vi "HandleXMLMapping.vi"(8 "error in (no error)":errorcluster, 10 "String":string, 11 "Node Ptr":T1 format="%.0x") -> (0 "error out":errorcluster, 3 "Node Ptr Out":T1 format="%.0x")   [LabVIEW 2024, in "Embedded TDMS Logger System Explorer.lvlib"]
doc: "Given an XML description of Sources and Destinations, creates these mappings in the System Definition."
uses:
  Embedded TDMS Logger System Explorer.lvlib
  <vilib>/NI VeriStand/Custom Device API/Custom Device Item Ref.ctl
  NationalInstruments.VeriStand.SystemDefinitionAPI
  NationalInstruments.VeriStand
  <vilib>/regexp/Match Regular Expression.xnode
  <vilib>/NI VeriStand/Custom Device API/Custom Device API.lvlib
panel:
  out "Array 3":string[](array[string])
  out "Array 2":i32[](array[numeric])
  out "Array":bool[](array[boolean])
  out "AddChannelMappings":bool
  out "Destinations":string[](array[string])
  out "Sources":string[](array[string])
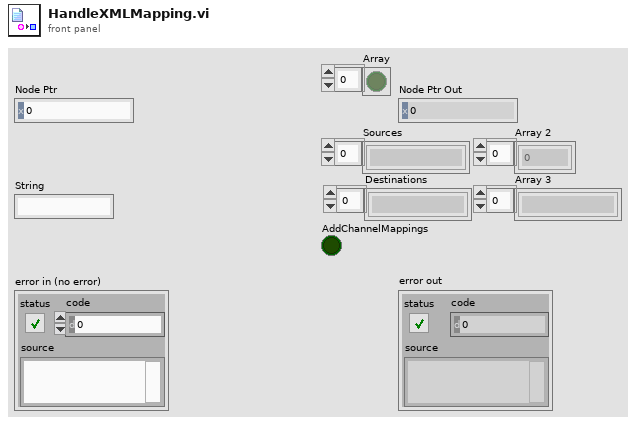
[diagram p1: front panel]
types:
  T1 = typedef "Custom Device API.lvlib/Custom Device Item Ref.ctl" = u64
  T2 = typedef "Custom Device API.lvlib/Custom Device Pointer.ctl" = refnum<k24>
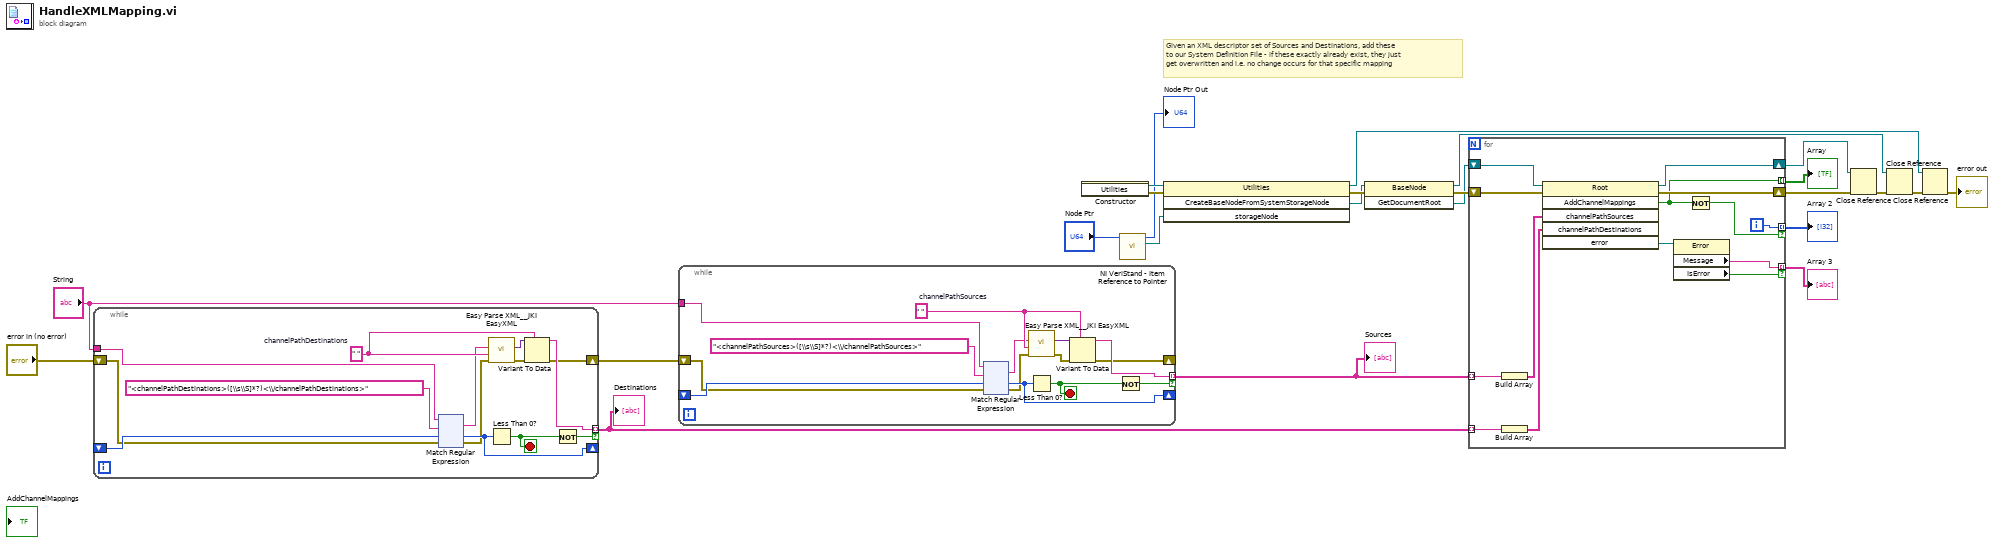
[diagram p0: block diagram]
diagram:
  # "Given an XML descriptor set of Sources and Destinations, add these\nto our System Definition File - if these exactly already exist, they just\nget overwritten and i.e. no change occurs for that specific mapping"
  n1 = while {
    shift-right: [w37] -> _
    shift-left: _ -> [w36]
    tunnel: "String" -> [w32]
    tunnel: [w31] -> w6 mode=indexing if=w28
    shift-right: [w26] -> w4
    shift-left: "error in (no error)" -> [w25]
    stop <- w27 stop-if-true
    w30 = " "  # channelPathDestinations
    n2 = xnode "Match Regular Expression"("input string"=w32, "regular expression"="<channelPathDestinations>([\\s\\S]*?)<\\/channelPathDestinations>" ("format string"), "offset (0)"=w36, "error in"=w25) -> ("whole match"=w29:string, "offset past match"=w37:i32, "error out"=w33:errorcluster)  [unwired: 2 in, 2 out]
    n3 = call <vilib>:"Easy Parse XML__JKI EasyXML.vi"("error in (no error)"=w33, "LabVIEW Data (Type)"=w30, "XML String"=w29) -> ("error out"=w35:errorcluster, "LabVIEW Data"=w34:variant)  [unwired: 7 in]
    n4 = Less Than 0?(x=w37) -> (x < 0?=w27:bool)
    n5 = Variant To Data(error in=w35, type=w30, Variant=w34) -> (data=w31:string, error out=w26:errorcluster)
    n6 = Not(x=w27) -> (.not. x?=w28:bool)
  }
  "Destinations" <- w6
  n7 = while {
    shift-right: [w168] -> _
    shift-left: _ -> [w167]
    tunnel: "String" -> [w163]
    tunnel: [w162] -> w5 mode=indexing if=w159
    shift-right: [w157] -> _
    shift-left: w4 -> [w156]
    stop <- w158 stop-if-true
    w161 = " "  # channelPathSources
    n8 = xnode "Match Regular Expression"("input string"=w163, "regular expression"="<channelPathSources>([\\s\\S]*?)<\\/channelPathSources>" ("format string"), "offset (0)"=w167, "error in"=w156) -> ("whole match"=w160:string, "offset past match"=w168:i32, "error out"=w164:errorcluster)  [unwired: 2 in, 2 out]
    n9 = call <vilib>:"Easy Parse XML__JKI EasyXML.vi"("error in (no error)"=w164, "LabVIEW Data (Type)"=w161, "XML String"=w160) -> ("error out"=w166:errorcluster, "LabVIEW Data"=w165:variant)  [unwired: 7 in]
    n10 = Less Than 0?(x=w168) -> (x < 0?=w158:bool)
    n11 = Variant To Data(error in=w166, type=w161, Variant=w165) -> (data=w162:string, error out=w157:errorcluster)
    n12 = Not(x=w158) -> (.not. x?=w159:bool)
  }
  "Sources" <- w5
  n13 = constructor class="Utilities"() -> (reference out=w12:refnum<k24>, error out=w13:errorcluster)  [unwired: 3 in, 1 out]
  n14 = call <vilib>:"NI VeriStand - Item Reference to Pointer.vi"("Item Ref in"="Node Ptr") -> ("Node Pointer"=w16:T2, "Item Ref out"=→"Node Ptr Out":T1)  [unwired: 7 in, 2 out]
  n15 = invoke class="Utilities" method="CreateBaseNodeFromSystemStorageNode"(reference=w12, error in=w13, "storageNode"=w16) -> (reference out=w23:refnum<k24>, error out=w15:errorcluster, "CreateBaseNodeFromSystemStorageNode"=w14:refnum<k24>)  [unwired: 1 in, 1 out]
  n16 = invoke class="BaseNode" method="GetDocumentRoot"(reference=w14, error in=w15) -> (reference out=w22:refnum<k24>, error out=w24:errorcluster, "GetDocumentRoot"=w10:refnum<k24>)  [unwired: 1 in]
  n17 = for {
    tunnel: w6 -> [w296] mode=indexing
    tunnel: w5 -> [w295] mode=indexing
    shift-right: [w298] -> w20
    shift-left: w24 -> [w300]
    shift-right: [w299] -> w21
    shift-left: w10 -> [w297]
    tunnel: [w291] -> w3 mode=indexing
    tunnel: [w292] -> w2 mode=indexing if=w290
    tunnel: [w288] -> w1 mode=indexing if=w287
    i -> [w292]
    n18 = Build Array(w295) -> (w294:string[])
    n19 = Build Array(w296) -> (w293:string[])
    n20 = invoke class="Root" method="AddChannelMappings"(reference=w297, error in=w300, "channelPathSources"=w294, "channelPathDestinations"=w293) -> (reference out=w299:refnum<k24>, error out=w298:errorcluster, "AddChannelMappings"=w291:bool, "error"=w289:refnum<k24>)  [unwired: 2 in, 2 out]
    n21 = property class="Error"(reference=w289) -> ("Message"=w288:string, "IsError"=w287:bool)  [unwired: 1 in, 2 out]
    n22 = Not(x=w291) -> (.not. x?=w290:bool)
  }
  "Array" <- w3
  "Array 2" <- w2
  "Array 3" <- w1
  n23 = Close Reference(reference=w21, error in (no error)=w20) -> (error out=w18:errorcluster)
  n24 = Close Reference(reference=w22, error in (no error)=w18) -> (error out=w19:errorcluster)
  n25 = Close Reference(reference=w23, error in (no error)=w19) -> (error out=→"error out":errorcluster)
